vi "Configure Resolution.vi"(8 "error in (no error)":errorcluster, 10 "Resolution":i32, 11 "PM-EMP in":refnum<class "PM-EMP.lvclass">) -> (0 "error out":errorcluster, 3 "PM-EMP out":refnum<class "PM-EMP.lvclass">)   [LabVIEW 2020, in "PM-EMP.lvclass"]
uses:
  PM-EMP.lvclass
  C:/Sandbox/Git_Sandbox/WiSpry Test Framework source code (LV20)/WiSpry Test Framework/Instruments/Instrument.lvclass
  Instrument.lvclass/Instrument.ctl
  Instrument.lvclass
panel:
  out "resulting string":string
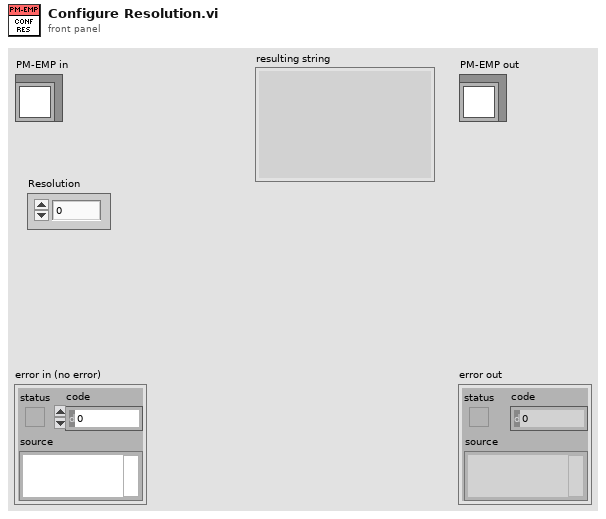
[diagram p1: front panel]
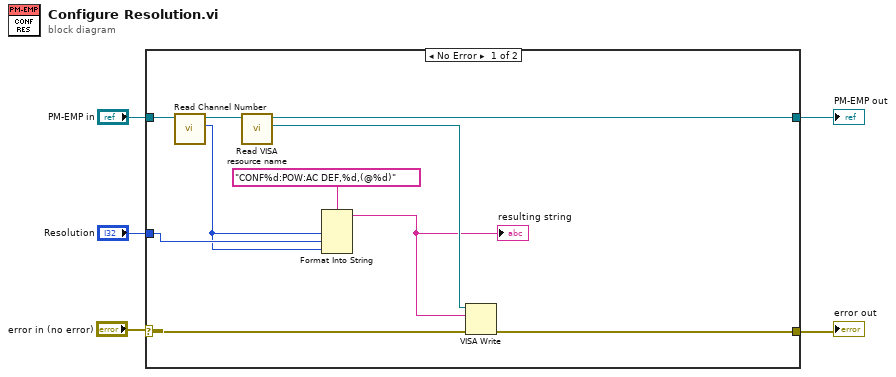
[diagram p0: block diagram]
diagram:
  n1 = case shown="No Error" "error in (no error)" {
    selector: "error in (no error)" -> [w11 w17]
    tunnel: [w10 w17] -> w4
    tunnel: "PM-EMP in" -> [w8 w16]
    tunnel: [w14 w16] -> w2
    tunnel: "Resolution" -> [w9 _]
    frame No Error {
      n2 = call-dynamic "Read Channel Number.vi"("Power Meter in"=w8) -> ("Channel Number"=w6:u8, "Power Meter out"=w7:refnum<class "PM-EMP.lvclass">)  [unwired: 9 in]
      n3 = call "Read VISA resource name.vi"("Instrument in"=w7) -> ("VISA resource name"=w15:refnum<visa-resource-name>, "Instrument out"=w14:refnum<class "PM-EMP.lvclass">)  [unwired: 9 in]
      n4 = Format Into String(format string="CONF%d:POW:AC DEF,%d,(@%d)", w6, w9, w6) -> (resulting string=w12:string)  [unwired: 2 in, 1 out]
      "resulting string" <- w12
      n5 = VISA Write(VISA resource name=w15, write buffer=w12, error in (no error)=w11) -> (error out=w10:errorcluster)  [unwired: 2 out]
    }
    frame Error {
    }
  }
  "error out" <- w4
  "PM-EMP out" <- w2
